vi "Construct.vi"(7 "Serial Configuration":T1, 10 "station":u8, 11 "series":i32(ring)=1 items=["AM", "H3U", "H5U"]) -> (3 "MelsecMcNet out":refnum<class "InovanceSerial.lvclass">)   [LabVIEW 2020, in "HslCommunication.lvlib" / "InovanceSerial.lvclass"]
uses:
  InovanceSerial.lvclass
  InovanceSerial.lvclass/InovanceSerial.ctl
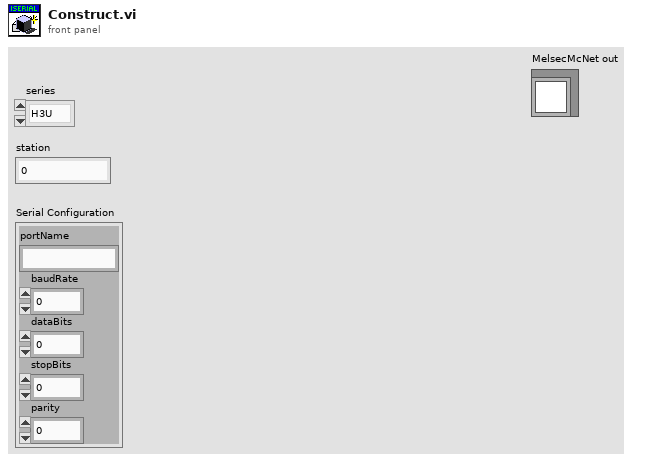
[diagram p1: front panel]
types:
  T1 = cluster{"portName":string, "baudRate":i32, "dataBits":i32, "stopBits":i32, "parity":i32}
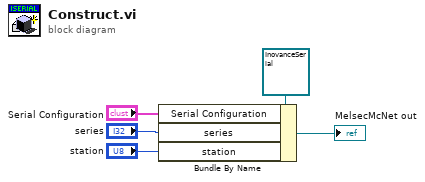
[diagram p0: block diagram]
diagram:
  n1 = Bundle By Name(cluster=refnum<class "InovanceSerial.lvclass"> refnum ("MelsecMcNet in"), "Serial Configuration"="Serial Configuration", "series"="series", "station"="station") -> (→"MelsecMcNet out":refnum<class "InovanceSerial.lvclass">)
